vi "COMANDOS.vi"() -> ()   [LabVIEW 2020]
panel:
  out "descripcion":string[](array[string])
  in  "Process Stop Button":bool
  in  "ENVIAR":bool
  in  "ingreso":string
  out "MONITOR":string
  out "GPS":bool
  out "respuestas":string[](array[string])
  out "comandos":string[](array[string])
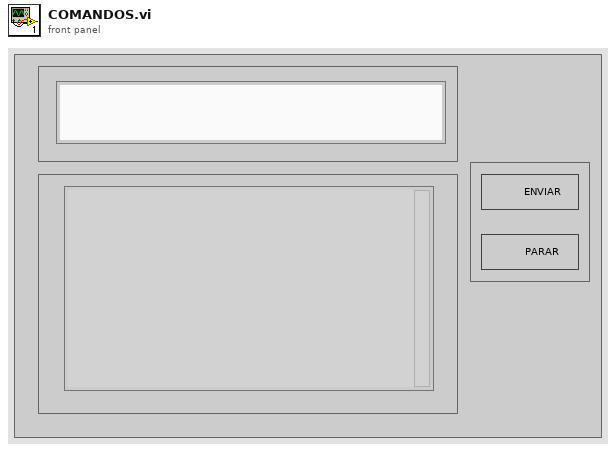
[diagram p1: front panel]
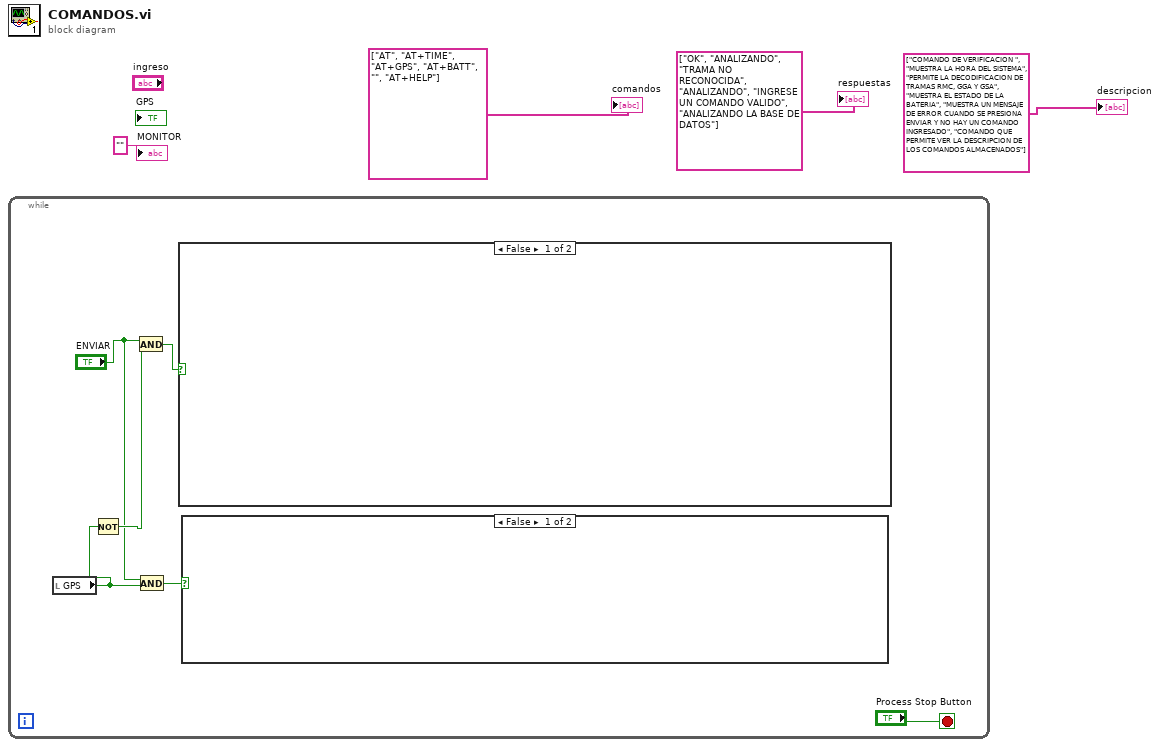
[diagram p0: block diagram]
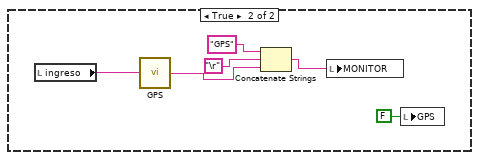
[diagram p2: hidden frame]
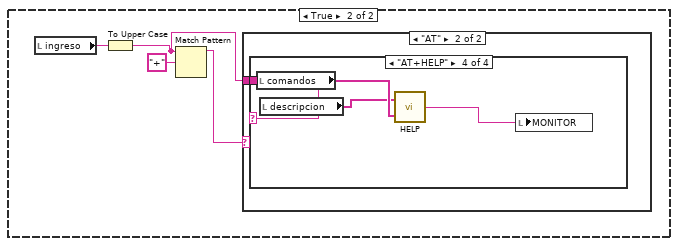
[diagram p3: hidden frame]
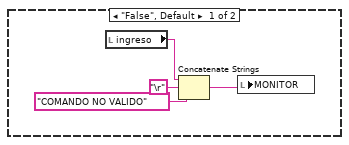
[diagram p4: hidden frame]
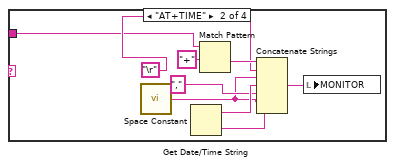
[diagram p6: hidden frame]
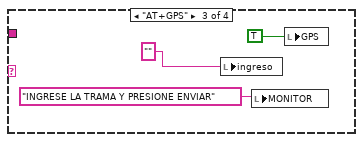
[diagram p7: hidden frame]
diagram:
  n1 = while {
    stop <- "Process Stop Button" stop-if-true
    n2 = local read "GPS"() -> (w8:bool)
    n3 = Not(x=w8) -> (.not. x?=w7:bool)
    n4 = And(x="ENVIAR", y=w7) -> (x .and. y?=w9:bool)
    n5 = And(x="ENVIAR", y=w8) -> (x .and. y?=w10:bool)
    n6 = case shown="False" w9 {
      frame False {
      }
      frame True {
        n7 = local read "ingreso"() -> (w18:string)
        n8 = To Upper Case(1:w18) -> (0:w17:string)
        n9 = Match Pattern(string=w17, regular expression="+") -> (before substring=w19:string)  [unwired: 1 in, 3 out]
        n10 = case shown="\"AT\"" w19 {
          tunnel: w17 -> [_ w25]
          frame "False", Default {
            n11 = local read "ingreso"() -> (w23:string)
            n12 = Concatenate Strings(w23, "\r", "COMANDO NO VALIDO" ("string")) -> (w24:string)
            n13 = local write "MONITOR"(w24) -> ()
          }
          frame "AT" {
            n14 = case shown="\"AT+HELP\"" w25 {
              tunnel: w25 -> [_ w26 _ _]
              frame "False", Default {
              }
              frame "AT+TIME" {
                n15 = call <vilib>:"Space Constant.vi"() -> ("String"=w29:string)
                n16 = Get Date/Time String() -> (date string=w32:string, time string=w28:string)  [unwired: 3 in]
                n17 = Match Pattern(string=w26, regular expression="+") -> (after substring=w34:string)  [unwired: 1 in, 3 out]
                n18 = Concatenate Strings(w34, "\r", w29, w32, "," ("string"), w29, w28) -> (w27:string)
                n19 = local write "MONITOR"(w27) -> ()
              }
              frame "AT+GPS" {
                n20 = local write "ingreso"("") -> ()
                n21 = local write "MONITOR"("INGRESE LA TRAMA Y PRESIONE ENVIAR" ("MONITOR")) -> ()
                n22 = local write "GPS"(TRUE ("AUX GPS")) -> ()
              }
              frame "AT+HELP" {
                n23 = local read "comandos"() -> (w39:string[])
                n24 = local read "descripcion"() -> (w38:string[])
                n25 = call "HELP.vi"("comando"=w39, "descripcion"=w38) -> ("MENSAJE"=w40:string)
                n26 = local write "MONITOR"(w40) -> ()
              }
            }
          }
        }
      }
    }
    n27 = case shown="False" w10 {
      frame False {
      }
      frame True {
        n28 = local read "ingreso"() -> (w16:string)
        n29 = call "GPS.vi"("Ingrese la trama"=w16) -> ("MENSAJE"=w15:string)
        n30 = Concatenate Strings("GPS", "\r", w15) -> (w14:string)
        n31 = local write "MONITOR"(w14) -> ()
        n32 = local write "GPS"(FALSE ("GPS")) -> ()
      }
    }
  }
  "comandos" <- string[] ["AT", "AT+TIME", "AT+GPS", "AT+BATT", "", "AT+HELP"]
  "respuestas" <- string[] ["OK", "ANALIZANDO", "TRAMA NO RECONOCIDA", "ANALIZANDO", "INGRESE UN COMANDO VALIDO", "ANALIZANDO LA BASE DE DATOS"]
  "MONITOR" <- "" ("MONITOR")
  "descripcion" <- string[] ["COMANDO DE VERIFICACION ", "MUESTRA LA HORA DEL SISTEMA", "PERMITE LA DECODIFICACION DE TRAMAS RMC, GGA Y GSA", "MUESTRA EL ESTADO DE LA BATERIA", "MUESTRA UN MENSAJE DE ERROR CUANDO SE PRESIONA ENVIAR Y NO HAY UN COMANDO INGRESADO", "COMANDO QUE PERMITE VER LA DESCRIPCION DE LOS COMANDOS ALMACENADOS"]
